vi "requestmessage.vi"(2 "error in (no error)":errorcluster, 3 "lockout_key":string, 4 "request content":string, 5 "msgop":i32(ring) items=["0"=0, "1"=1, "6"=6, "7"=7, "8"=8, "9"=9]) -> (0 "error out":errorcluster, 1 "body":string)   [LabVIEW 2016]
doc: "Format the message to follow dripline standard"
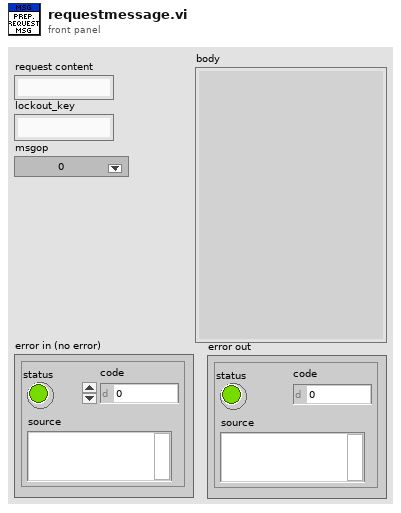
[diagram p1: front panel]
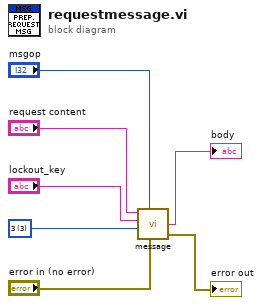
[diagram p0: block diagram]
diagram:
  w4 = 3 items=["2"=2, "3"=3, "4"=4] ("msgtype")
  n1 = call "message.vi"("input json string"="request content", "msgop"="msgop", "lockout_key"="lockout_key", "msgtype"=w4, "error in (no error)"="error in (no error)") -> ("body"=→"body":string, "error out"=→"error out":errorcluster)  [unwired: 2 in]
